vi "Alert.vi"   [LabVIEW 2019]
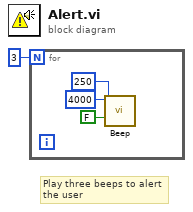
[diagram p0: block diagram]
diagram:
  # "Play three beeps to alert\nthe user"
  n1 = for {
    N: 3 -> [_]
    n2 = call <vilib>:"Beep.vi"("use system alert? (T)"=FALSE, "duration (msec)"=u32 250, "frequency (Hz)"=u32 4000) -> ()  [unwired: 9 in]
  }
